vi "LV SciSDK DIGITIZER START.vi"(0 "Digitizer Name":string, 1 "Acq mode":string(combo)="blocking", 2 "Timeout":i32=100, 3 "High performance":string(combo)="false", 5 "Enabled channels":u32=1, 7 "Acq len":u32=1024, 9 "Board Handle In":T1, 11 "error in (no error)":errorcluster) -> (8 "Digitizer Handle Out":T2, 10 "Board Handle Out":T1, 15 "error out":errorcluster)   [LabVIEW 2021]
uses:
  SciSDK_Labview.lvlib
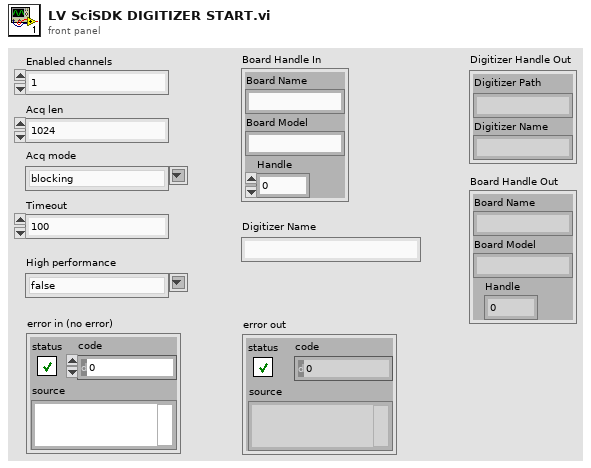
[diagram p1: front panel]
types:
  T1 = cluster{"Board Name":string, "Board Model":string, "Handle":u64}
  T2 = cluster{"Digitizer Path":string, "Digitizer Name":string}
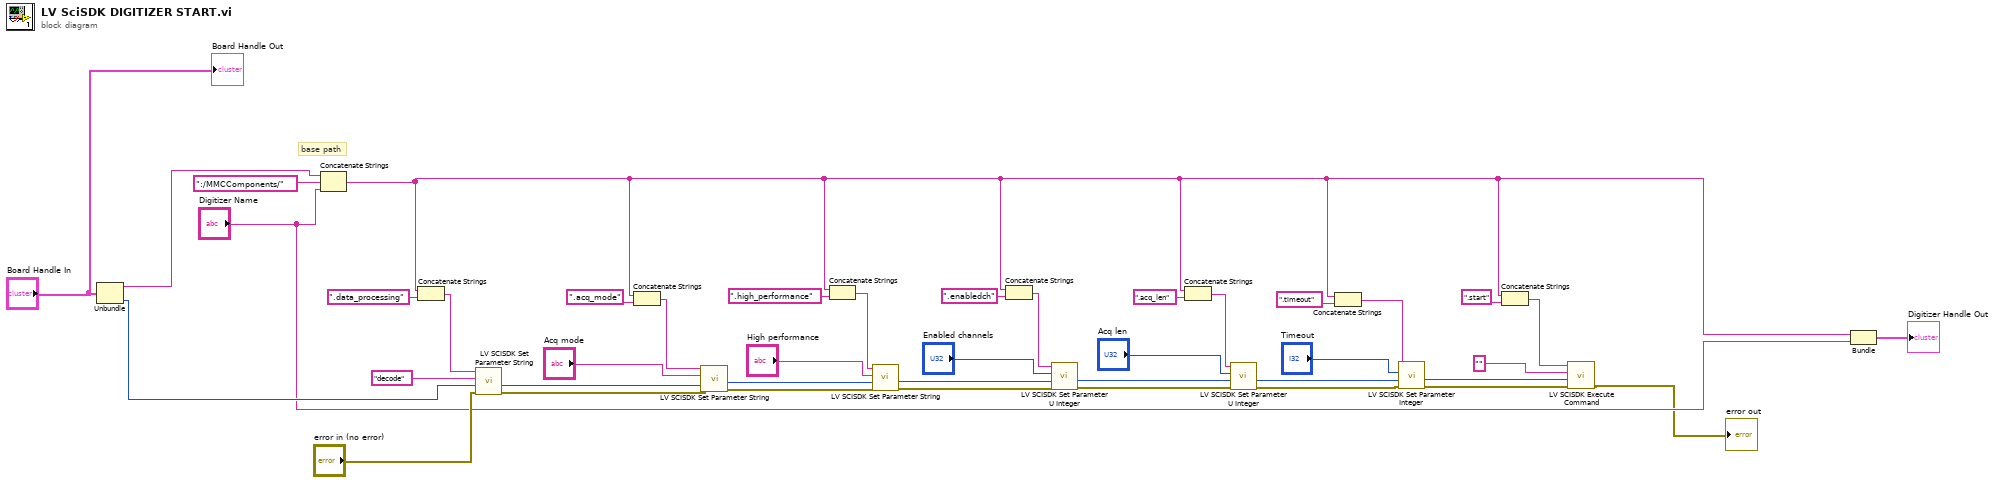
[diagram p0: block diagram]
diagram:
  # "base path"
  n1 = Unbundle("Board Handle In") -> ("Board Name"=w41:string, "Handle"=w37:u64)  [unwired: 1 out]
  n2 = Concatenate Strings(w41, ":/MMCComponents/" ("string"), "Digitizer Name") -> (w2:string)
  n3 = Concatenate Strings(w2, ".data_processing" ("string")) -> (w39:string)
  n4 = call "LV SCISDK Set Parameter String.vi"("error in (no error)"="error in (no error)", "handle"=w37, "value"="decode", "Path"=w39) -> ("error out"=w35:errorcluster, "handle out"=w26:u64)  [unwired: 5 in, 1 out]
  n5 = Concatenate Strings(w2, ".acq_mode" ("string")) -> (w28:string)
  n6 = call "LV SCISDK Set Parameter String.vi"("error in (no error)"=w35, "handle"=w26, "value"="Acq mode", "Path"=w28) -> ("error out"=w34:errorcluster, "handle out"=w25:u64)  [unwired: 5 in, 1 out]
  n7 = Concatenate Strings(w2, ".high_performance" ("string")) -> (w23:string)
  n8 = call "LV SCISDK Set Parameter String.vi"("error in (no error)"=w34, "handle"=w25, "value"="High performance", "Path"=w23) -> ("error out"=w22:errorcluster, "handle out"=w21:u64)  [unwired: 5 in, 1 out]
  n9 = Concatenate Strings(w2, ".enabledch" ("string")) -> (w20:string)
  n10 = call "LV SCISDK Set Parameter U Integer.vi"("error in (no error)"=w22, "handle"=w21, "value"="Enabled channels", "Path"=w20) -> ("error out"=w18:errorcluster, "handle out"=w17:u64)  [unwired: 5 in, 1 out]
  n11 = Concatenate Strings(w2, ".acq_len" ("string")) -> (w15:string)
  n12 = call "LV SCISDK Set Parameter U Integer.vi"("error in (no error)"=w18, "handle"=w17, "value"="Acq len", "Path"=w15) -> ("error out"=w14:errorcluster, "handle out"=w12:u64)  [unwired: 5 in, 1 out]
  n13 = Concatenate Strings(w2, ".timeout" ("string")) -> (w11:string)
  n14 = call "LV SCISDK Set Parameter Integer.vi"("error in (no error)"=w14, "handle"=w12, "value"="Timeout", "Path"=w11) -> ("error out"=w6:errorcluster, "handle out"=w5:u64)  [unwired: 5 in, 1 out]
  n15 = Concatenate Strings(w2, ".start" ("string")) -> (w7:string)
  n16 = call "LV SCISDK Execute Command.vi"("error in (no error)"=w6, "handle"=w5, "value"="", "Path"=w7) -> ("error out"=→"error out":errorcluster)  [unwired: 5 in, 2 out]
  n17 = Bundle(w2, "Digitizer Name"="Digitizer Name") -> (→"Digitizer Handle Out":cluster{string, "Digitizer Name":string})  [unwired: 1 in]
  "Board Handle Out" <- "Board Handle In"
